vi "oax_gsOrbit Plot.vi"() -> ()   [LabVIEW 2017]
doc: "This is Order Analysis Toolkit demo VI."
uses:
  <vilib>/addons/Sound and Vibration/Order Analysis/Tach Process/SoundVib_TachProcess.lvlib
  <vilib>/addons/Sound and Vibration/Order Analysis/Resample Order Tracking/SoundVib_OrderTracking.lvlib
  <vilib>/Waveform/WDTOps.llb/WDT Waveform Duration DBL.vi
  <vilib>/addons/Sound and Vibration/Order Analysis/Utility/SoundVib_OAUtility.lvlib
  <vilib>/addons/Sound and Vibration/Order Analysis/Data Presentation/SoundVib_MCMDisplay.lvlib
  <vilib>/addons/Sound and Vibration/Order Analysis/Data Presentation/SVX Orbit and Timebase Plot (Unfiltered).vi
  <vilib>/addons/Sound and Vibration/Order Analysis/Utility/OAT AC DC Separation (N Channels).vi
  <vilib>/addons/Sound and Vibration/Order Analysis/Data Presentation/SVX Orbit and Timebase Plot (Filtered) (N Ch - 1 Order).vi
  <vilib>/addons/_XControls/Orbit Plot/SVX Orbit.xctl
panel:
  out "Orbit Plot":T1(xcontrol)
  in  "bandwidth [order]":dbl format="%.2f"
  in  "max order (auto)":dbl
  in  "plot type":u16(ring)=1 items=["unfiltered plot", "filtered plot"]
  in  "samples/rev wanted":i32=64
  out "orbit precession direction":u16(ring) items=["forward", "backward"]
  in  "order to display":dbl=1.0 format="%.2f"
  in  "channel settings":T2={"shaft rotating\ndirection"=0, "probe angles [deg]"={"X"=0, "Y"=90}} {"probe angles [deg]"."Y" max=360 step=1; "probe angles [deg]"."X" max=360 step=1; "shaft rotating\ndirection" items=["CCW", "CW"]}
  in  "orbit plot display revolutions":cluster{"duration [rev]":dbl}={"duration [rev]"=1.0} {"duration [rev]" format="%.2f"}
  in  "STOP":bool
  in  "Select Data":i32(listbox)
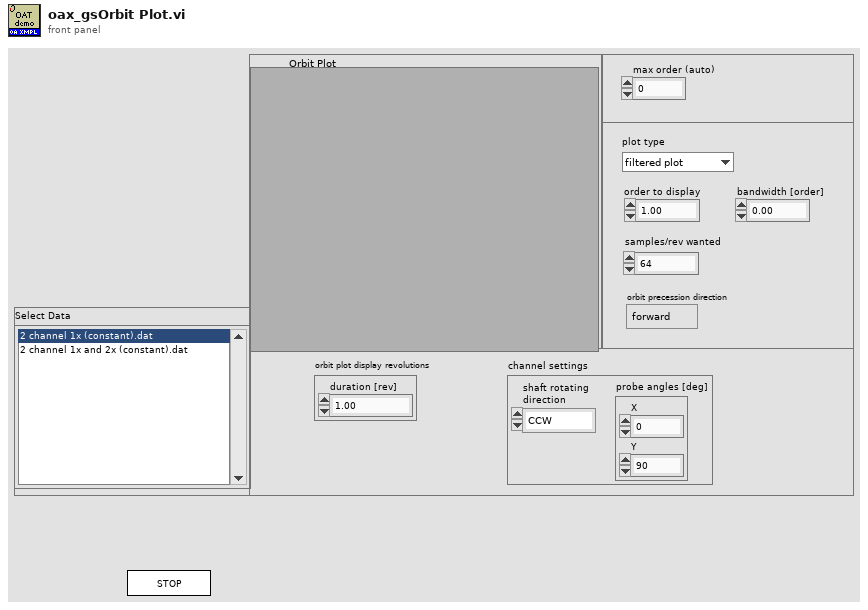
[diagram p1: front panel]
types:
  T1 = cluster{"probe x":dbl[], "probe y":dbl[], "reference":dbl[], "plot type":enum16{"Filtered Plot", "Unfiltered Plot"}, "attribute":variant}[][]
  T2 = cluster{"shaft rotating\ndirection":u16, "probe angles [deg]":cluster{"X":u32, "Y":u32}}
  T3 = cluster{"dB on? (T)":bool, "unwrap phase? (T)":bool, "unit in degree? (T)":bool}
  T4 = typedef "SoundVib_TachProcess.lvlib/speed profile.ctl" = cluster{"time [s]":dbl[], "speed [RPM]":dbl[]}
  T5 = typedef "svc_Resampled Channel Info.ctl" = cluster{"channel name":string, "description":string, " channel info":T6}
  T6 = typedef "svc_Channel Info.ctl" = cluster{"sensor sensitivity":dbl, "engineering units":T7, "dB reference":dbl, "custom label":string, "weighting filter":T8, "pregain":dbl}
  T7 = typedef "svc_Engineering Units Text Ring.ctl" = u16
  T8 = typedef "svc_Weighting Filter Text Ring.ctl" = u16
  T9 = typedef "OAT Position Info.ctl" = cluster{"positions [s]":dbl[], "samples/rev":dbl}
  T10 = cluster{"shaft rotating\ndirection":u16, "X":u32, "pair":u16}
  T11 = cluster{"shaft rotating\ndirection":u16, "Y":u32, "pair":u16}
  T12 = cluster{"shaft rotating\ndirection":u16, "Y":u32, "pair":u16}[]
  T13 = cluster{"time/rev/rpm":dbl[], "magnitude":dbl[]}[][]
  T14 = typedef "svc_Spectrum Info.ctl" = cluster{"channel name":string, "description":string, "x-axis units":T15, "spectral info":cluster{"spectrum type":T16, "linear/dB":enum16{"linear", "dB"}, "window":u16, "window size":i32, "FFT size":i32}, "engineering units":T7, "custom label":string, "dB reference [EU]":dbl, "peak units":enum16{"rms", "peak", "peak-peak"}, "weighting filter":T8, "spectral density?":bool, "unit label":string, "spectrum skewed?":bool, "complimentary spectrum units":T17}
  T15 = typedef "svc_X-Axis Units.ctl" = u16
  T16 = typedef "svc_Spectrum Type.ctl" = enum16{"FFT Spectrum [complex]", "Amplitude [Magnitude]", "Power [Magnitude^2]", "Cross Spectrum [complex]", "Frequency Response [Complex]"}
  T17 = typedef "svc_Complimentary Spectrum Units.ctl" = enum16{"none", "radians", "degrees", "cycles", "imaginary"}
  T18 = cluster{"time/rev/rpm":dbl[], "magnitude":dbl[]}[]
  T19 = cluster{"pulse / rev":i32, "threshold (auto)":dbl, "slope (Rising)":u16}
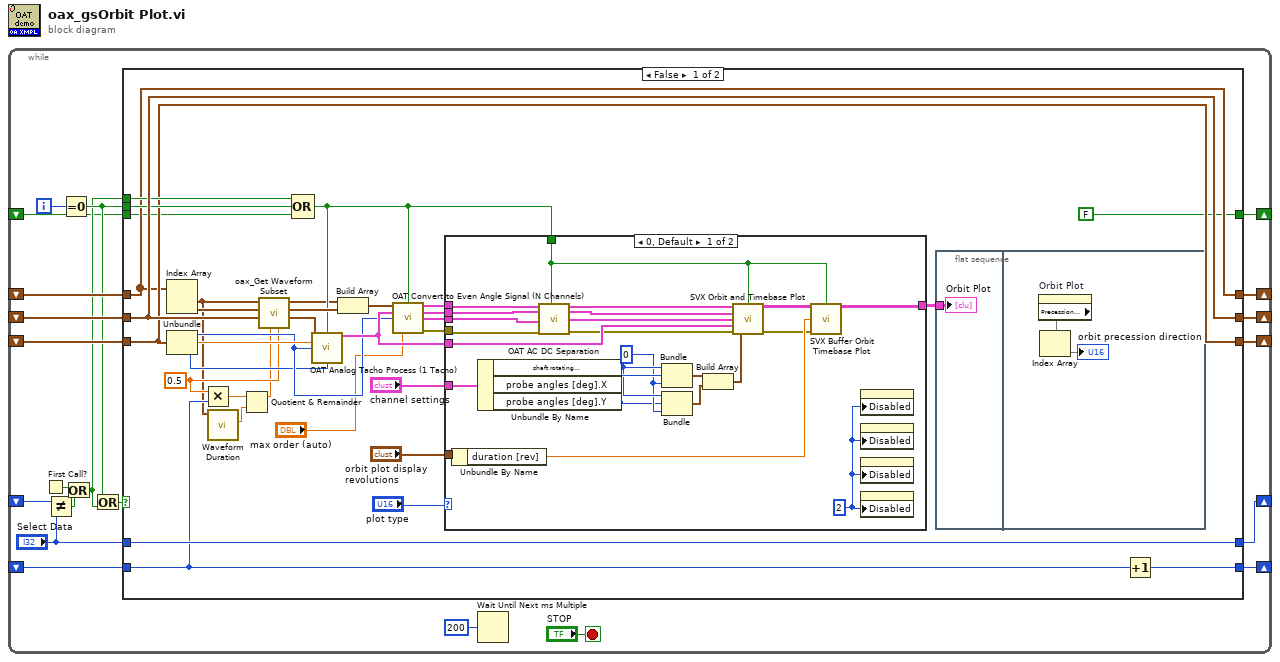
[diagram p0: block diagram]
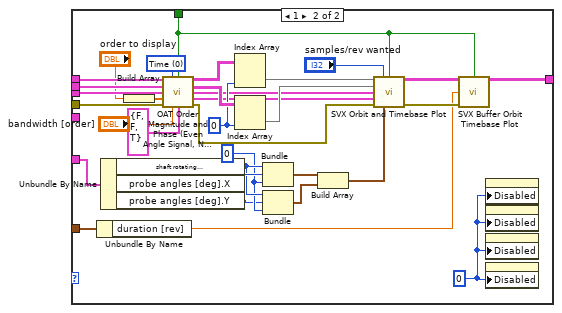
[diagram p2: hidden frame]
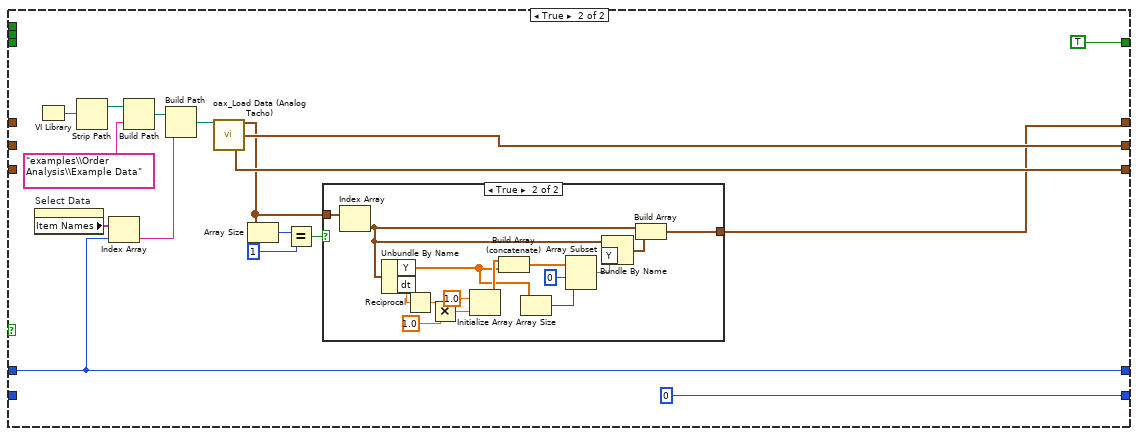
[diagram p3: hidden frame]
diagram:
  n1 = while {
    shift-right: [w17] -> _
    shift-left: _ -> [w18]
    shift-right: [w15] -> _
    shift-left: _ -> [w21]
    shift-right: [w14] -> _
    shift-left: _ -> [w19]
    shift-right: [w13] -> _
    shift-left: _ -> [w12]
    shift-right: [w3] -> _
    shift-left: _ -> [w4]
    shift-right: [w2] -> _
    shift-left: _ -> [w1]
    i -> [w11]
    stop <- "STOP" stop-if-true
    n2 = First Call?() -> (First Call?: T/F=w7:bool)
    n3 = Not Equal?(x=w18, y="Select Data") -> (x != y?=w6:bool)
    n4 = Equal To 0?(x=w11) -> (x = 0?=w10:bool)
    n5 = Or(x=w7, y=w6) -> (x .or. y?=w5:bool)
    n6 = Or(x=w10, y=w5) -> (x .or. y?=w9:bool)
    n7 = case shown="False" w9 {
      tunnel: w21 -> [w34 _]
      tunnel: w19 -> [w53 _]
      tunnel: [w54 w131] -> w17
      tunnel: "Select Data" -> [w54 w131]
      tunnel: [w34 w116] -> w15
      tunnel: [w53 w129] -> w14
      tunnel: [w45 w128] -> w13
      tunnel: w12 -> [w45 _]
      tunnel: w5 -> [w50 _]
      tunnel: w10 -> [w49 _]
      tunnel: w4 -> [w39 _]
      tunnel: [w41 0] -> w3
      tunnel: [FALSE TRUE] -> w2
      tunnel: w1 -> [w33 _]
      frame False {
        w40 = 0.5 ("y")
        n8 = Index Array(array=w34) -> (element #1=w38:waveform(dbl), element #2=w46:waveform(dbl))  [unwired: 2 in]
        n9 = Unbundle(w45) -> ("pulse / rev"=w43:i32, "threshold (auto)"=w44:dbl, "slope (Rising)"=w42:u16)
        n10 = Multiply(x=w40, y=w39) -> (x*y=w36:dbl)
        n11 = call-poly <vilib>:"Waveform Duration.vi"("waveform in"=w38) -> ("duration"=w37:dbl)  [unwired: 8 in, 2 out]
        n12 = Quotient & Remainder(x=w36, y=w37) -> (x-y*floor(x/y)=w35:dbl)  [unwired: 1 out]
        n13 = call <vilib>:"oax_Get Waveform Subset.vi"("duration"=w40, "start index"=w35, "Tach Signal"=w53, "Vibration Signal Y"=w46, "Vibration Signal X"=w38) -> ("Tach Signal out"=w51:waveform(dbl), "Vibration Signal Y out"=w52:waveform(dbl), "Vibration Signal X out"=w47:waveform(dbl))  [unwired: 3 in, 1 out]
        n14 = Compound Arithmetic op=OR(w50, w49, w33) -> (w48:bool)
        n15 = call <vilib>:"OAT Analog Tacho Process (1 Tacho).vi"("analog tacho signal"=w51, "reset? (F)"=w48, "threshold (auto)"=w44, "pulse/revolution (1)"=w43, "slope (Rising)"=w42) -> ("speed profile"=w55:T4)  [unwired: 6 in, 4 out]
        n16 = Build Array(w47, w52) -> (w31:waveform(dbl)[])
        n17 = call <vilib>:"OAT Convert to Even Angle Signal (N Channels).vi"("scaled signals [EU]"=w31, "reset? (F)"=w48, "speed profile"=w55, "pulse/revolution (1)"=w43, "max order (auto)"="max order (auto)") -> ("even-angle signals"=w25:cluster{"r0":dbl, "dr":dbl, "Y":dbl[]}[], "even-angle channel info"=w24:T5[], "even-angle position info"=w23:T9, "error out"=w30:errorcluster)  [unwired: 6 in, 1 out]
        n18 = case shown="0, Default" "plot type" {
          tunnel: [w65 w87] -> w22
          tunnel: w25 -> [w79 w115]
          tunnel: w55 -> [w76 _]
          tunnel: w23 -> [w77 w113]
          tunnel: w24 -> [w78 w114]
          tunnel: w30 -> [w59 w112]
          tunnel: w48 -> [w64 w86]
          tunnel: "orbit plot display revolutions" -> [w63 w84]
          tunnel: "channel settings" -> [w74 w90]
          frame 0, Default {
            w82 = u8 2 ("Disabled")
            w71 = u16 0 ("pair")
            n19 = Unbundle By Name(w63) -> ("duration [rev]"=w62:dbl)
            n20 = Unbundle By Name(w74) -> ("shaft rotating\ndirection"=w72:u16, "probe angles [deg].X"=w73:u32, "probe angles [deg].Y"=w70:u32)
            n21 = call-poly <vilib>:"OAT AC DC Separation.vi"("even-angle signals"=w79, "even-angle channel info"=w78, "position info"=w77, "error in (no error)"=w59, "reset? (F)"=w64) -> ("even-angle AC signals"=w81:cluster{"r0":dbl, "dr":dbl, "Y":dbl[]}[], "dup even-angle channel info"=w80:T5[], "position info out"=w75:T9, "error out"=w60:errorcluster)  [unwired: 9 in, 2 out]
            n22 = Bundle("shaft rotating\ndirection"=w72, "X"=w73, "pair"=w71) -> (w69:T10)  [unwired: 1 in]
            n23 = Bundle("shaft rotating\ndirection"=w72, "Y"=w70, "pair"=w71) -> (w68:T11)  [unwired: 1 in]
            n24 = Build Array(w69, w68) -> (w67:T12)
            n25 = call-poly <vilib>:"SVX Orbit and Timebase Plot.vi"("even-angle signals"=w81, "reset? (F)"=w64, "even-angle channel info"=w80, "even-angle position info"=w75, "speed profile"=w76, "error in (no error)"=w60, "channel properties"=w67) -> ("orbit/timebase plot"=w66:T1, "error out"=w61:errorcluster)  [unwired: 5 in, 2 out]
            n26 = call <vilib>:"SVX Buffer Orbit Timebase Plot.vi"("orbit/timebase plot in"=w66, "reset? (F)"=w64, "buffer size (rev)"=w62, "error in (no error)"=w61) -> ("orbit/timebase plot out"=w65:T1)  [unwired: 10 in, 1 out]
            n27 = property on="bandwidth [order]" class="DigNum (strict)"("Disabled"=w82) -> ()  [unwired: 2 in, 2 out]
            n28 = property on="order to display" class="DigNum (strict)"("Disabled"=w82) -> ()  [unwired: 2 in, 2 out]
            n29 = property on="samples/rev wanted" class="DigNum (strict)"("Disabled"=w82) -> ()  [unwired: 2 in, 2 out]
            n30 = property on="orbit precession direction" class="Ring (strict)"("Disabled"=w82) -> ()  [unwired: 2 in, 2 out]
          }
          frame 1 {
            w105 = u8 0 ("Disabled")
            w94 = u16 0 ("pair")
            w108 = u16 0 items=["Time", "Revolution", "RPM"] ("X axis selection")
            w107 = 0 ("disabled index (col)")
            n31 = Unbundle By Name(w84) -> ("duration [rev]"=w83:dbl)
            n32 = Unbundle By Name(w90) -> ("shaft rotating\ndirection"=w95:u16, "probe angles [deg].X"=w96:u32, "probe angles [deg].Y"=w93:u32)
            n33 = Build Array("order to display") -> (w109:dbl[])
            n34 = call <vilib>:"OAT Order Magnitude and Phase (Even Angle Signal, N Channels).vi"("even-angle signals"=w115, "x-axis selection"=w108, "reset? (F)"=w86, "even-angle channel info"=w114, "even-angle position info"=w113, "orders to compute (1.0)"=w109, "error in (no error)"=w112, "bandwidth [order]"="bandwidth [order]", "view"=T3 {"dB on? (T)"=FALSE, "unwrap phase? (T)"=FALSE, "unit in degree? (T)"=TRUE}) -> ("magnitudes [RMS]"=w111:T13, "phases [phase lag]"=w110:cluster{"time/rev/rpm":dbl[], "phase":dbl[]}[][], "magnitude/phase position info"=w100:T9, "magnitudes info"=w99:T14[], "error out"=w97:errorcluster)  [unwired: 1 in, 1 out]
            n35 = Index Array(array=w111, index (col)=w107) -> (element=w102:T18)  [unwired: 1 in]
            n36 = Index Array(array=w110, index (col)=w107) -> (element=w101:cluster{"time/rev/rpm":dbl[], "phase":dbl[]}[])  [unwired: 1 in]
            n37 = Bundle("shaft rotating\ndirection"=w95, "X"=w96, "pair"=w94) -> (w92:T10)  [unwired: 1 in]
            n38 = Bundle("shaft rotating\ndirection"=w95, "Y"=w93, "pair"=w94) -> (w91:T11)  [unwired: 1 in]
            n39 = Build Array(w92, w91) -> (w89:T12)
            n40 = call-poly <vilib>:"SVX Orbit and Timebase Plot.vi"("magnitudes [RMS]"=w102, "samples/rev wanted"="samples/rev wanted", "reset? (F)"=w86, "phases [phase lag]"=w101, "magnitude/phase position info"=w100, "magnitudes info"=w99, "error in (no error)"=w97, "channel properties"=w89) -> ("orbit/timebase plot"=w88:T1, "error out"=w85:errorcluster)  [unwired: 4 in, 2 out]
            n41 = call <vilib>:"SVX Buffer Orbit Timebase Plot.vi"("orbit/timebase plot in"=w88, "reset? (F)"=w86, "buffer size (rev)"=w83, "error in (no error)"=w85) -> ("orbit/timebase plot out"=w87:T1)  [unwired: 10 in, 1 out]
            n42 = property on="bandwidth [order]" class="DigNum (strict)"("Disabled"=w105) -> ()  [unwired: 2 in, 2 out]
            n43 = property on="order to display" class="DigNum (strict)"("Disabled"=w105) -> ()  [unwired: 2 in, 2 out]
            n44 = property on="samples/rev wanted" class="DigNum (strict)"("Disabled"=w105) -> ()  [unwired: 2 in, 2 out]
            n45 = property on="orbit precession direction" class="Ring (strict)"("Disabled"=w105) -> ()  [unwired: 2 in, 2 out]
          }
        }
        n46 = flat-sequence {
          tunnel: w22 -> [w56]
          frame #0 {
            "Orbit Plot" <- w56
          }
          frame #1 {
            n47 = property on="Orbit Plot"() -> ("Precession Direcition"=w58)  [unwired: 2 in, 2 out]
            n48 = Index Array(array=w58) -> (element=→"orbit precession direction")  [unwired: 1 in]
          }
        }
        n49 = Increment(x=w39) -> (x+1=w41:i32)
      }
      frame True {
        n50 = property on="Select Data" class="LstBox (strict)"() -> ("Item Names"=w132:string[])  [unwired: 2 in, 2 out]
        n51 = VI Library() -> (path=w124:path)
        n52 = Strip Path(path=w124) -> (stripped path=w123:path)  [unwired: 1 out]
        n53 = Index Array(array=w132, index=w131) -> (element=w126:string)
        n54 = Build Path(base path=w123, name or relative path="examples\\Order Analysis\\Example Data") -> (appended path=w127:path)
        n55 = Build Path(base path=w127, name or relative path=w126) -> (appended path=w125:path)
        n56 = call <vilib>:"oax_Load Data (Analog Tacho).vi"("Data Path In"=w125) -> ("vibration data"=w117:waveform(dbl)[], "analog tacho signal"=w129:waveform(dbl), "tacho info"=w128:T19)  [unwired: 8 in, 4 out]
        n57 = Array Size(array=w117) -> (size(s)=w120:i32)
        n58 = Equal?(x=w120, y=1) -> (x = y?=w118:bool)
        n59 = case shown="True" w118 {
          tunnel: w117 -> [w133 w148]
          tunnel: [w133 w147] -> w116
          frame False {
          }
          frame True {
            n60 = Index Array(array=w148) -> (element=w146:waveform(dbl))  [unwired: 1 in]
            n61 = Unbundle By Name(w146) -> ("Y"=w135:dbl[], "dt"=w144:dbl)
            n62 = Reciprocal(x=w144) -> (1/x=w143:dbl)
            n63 = Multiply(x=w143, y=1.0) -> (x*y=w141:dbl)
            n64 = Initialize Array(1.0 ("element"), w141) -> (w137:dbl[])
            n65 = Build Array (concatenate)(w137, w135) -> (w139:dbl[])
            n66 = Array Size(array=w135) -> (size(s)=w136:i32)
            n67 = Array Subset(array=w139, index=0, length=w136) -> (w134:dbl[])
            n68 = Bundle By Name(cluster=w146, "Y"=w134) -> (w145:waveform(dbl))
            n69 = Build Array(w146, w145) -> (w147:waveform(dbl)[])
          }
        }
      }
    }
    n70 = Wait Until Next ms Multiple(millisecond multiple=u32 200) -> ()  [unwired: 1 out]
  }
